vi "RobotOpen.vi"(8 "error in (no error)":errorcluster, 11 "Robot Communication port name":refnum<visa-resource-name>="ASRL2::INSTR") -> (0 "error out":errorcluster, 3 "Robot Communication port name out":refnum<visa-resource-name>)   [LabVIEW 2017]
doc: "Open UART serial port and initilize iRobot."
uses:
  <vilib>/myRIO/Instrument Drivers/Onboard IO/UART/typedef/VISA Configuration.ctl
  <vilib>/Instr/_visa.llb/VISA Flush IO Buffer Mask.ctl
  <vilib>/Instr/_visa.llb/VISA Configure Serial Port (Instr).vi
  <vilib>/myRIO/Instrument Drivers/Onboard IO/UART/UART.lvlib
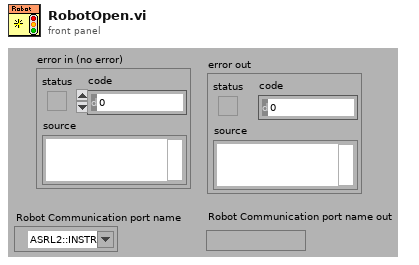
[diagram p1: front panel]
types:
  T1 = typedef "VISA Flush IO Buffer Mask.ctl" = u16
  T2 = typedef "UART.lvlib/VISA Configuration.ctl" = cluster{"baud rate (9600)":u32, "data bits (8)":u16, "parity (0:none)":enum16{"None", "Odd", "Even", "Mark", "Space"}, "stop bits (10: 1 bit)":u16, "flow control (0:none)":u16, "termination char\n(0xA = '\\n' = LF) ":u8, "Enable Termination\nChar (T)":bool, "timeout (10sec)":u32}
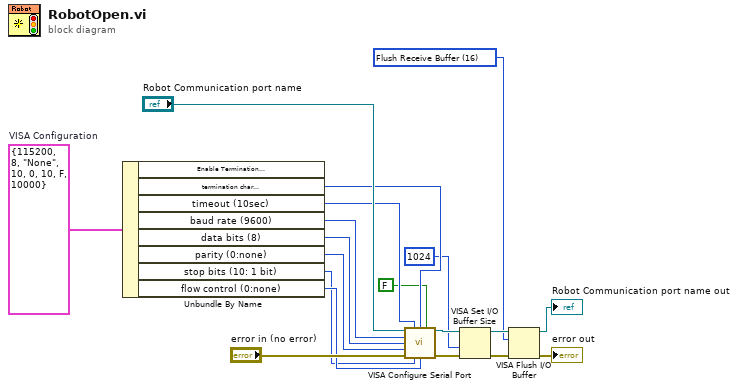
[diagram p0: block diagram]
diagram:
  w2 = T1 16 items=["Flush Receive Buffer"=16, "Write Transmit Buffer to Device"=32, "Flush Receive Buffer (No I/O)"=64, "Flush Transmit Buffer"=128] ("Mask")
  w15 = T2 {"baud rate (9600)"=115200, "data bits (8)"=8, "parity (0:none)"=enum."None", "stop bits (10: 1 bit)"=10, "flow control (0:none)"=0, "termination char\n(0xA = '\\n' = LF) "=10, "Enable Termination\nChar (T)"=FALSE, "timeout (10sec)"=10000}  # VISA Configuration
  n1 = Unbundle By Name(w15) -> ("termination char\n(0xA = '\\n' = LF)"=w14:u8, "timeout (10sec)"=w13:u32, "baud rate (9600)"=w8:u32, "data bits (8)"=w9:u16, "parity (0:none)"=w10:enum16{"None", "Odd", "Even", "Mark", "Space"}, "stop bits (10: 1 bit)"=w11:u16, "flow control (0:none)"=w12:u16)  [unwired: 1 out]
  n2 = call-poly "VISA Configure Serial Port"("VISA resource name"="Robot Communication port name", "timeout (10sec)"=w13, "termination char\n(0xA = '\\n' = LF)"=w14, "Enable Termination\nChar (T)"=FALSE ("Enable Termination\nChar (T)"), "baud rate (9600)"=w8, "data bits (8)"=w9, "parity (0:none)"=w10, "error in (no error)"="error in (no error)", "stop bits (10: 1 bit)"=w11, "flow control (0:none)"=w12) -> ("VISA resource name out"=w6:refnum<visa-resource-name>, "error out"=w5:errorcluster)  [unwired: 4 in]
  n3 = VISA Set I/O Buffer Size(VISA resource name=w6, size (4096)=u32 1024, error in (no error)=w5) -> (VISA resource name out=w3:refnum<visa-resource-name>, error out=w1:errorcluster)  [unwired: 1 in]
  n4 = VISA Flush I/O Buffer(VISA resource name=w3, mask (16)=w2, error in (no error)=w1) -> (VISA resource name out=→"Robot Communication port name out":refnum<visa-resource-name>, error out=→"error out":errorcluster)
